vi "SaveImage.vi"(6 "x":dbl, 7 "error in (no error)":errorcluster, 8 "in path":path, 9 "Snap":bool, 10 "Image In":T1) -> (0 "error out":errorcluster)   [LabVIEW 2017]
uses:
  <vilib>/vision/Image Controls.llb/IMAQ Image.ctl
  <vilib>/vision/driver/IMAQdx.llb/IMAQdx Acquisition Mode.ctl
  <vilib>/vision/driver/NI_Vision_Acquisition_Software.lvlib
panel:
  out "Image":T1(plugin-control)
  out "number (0 to 1)":dbl
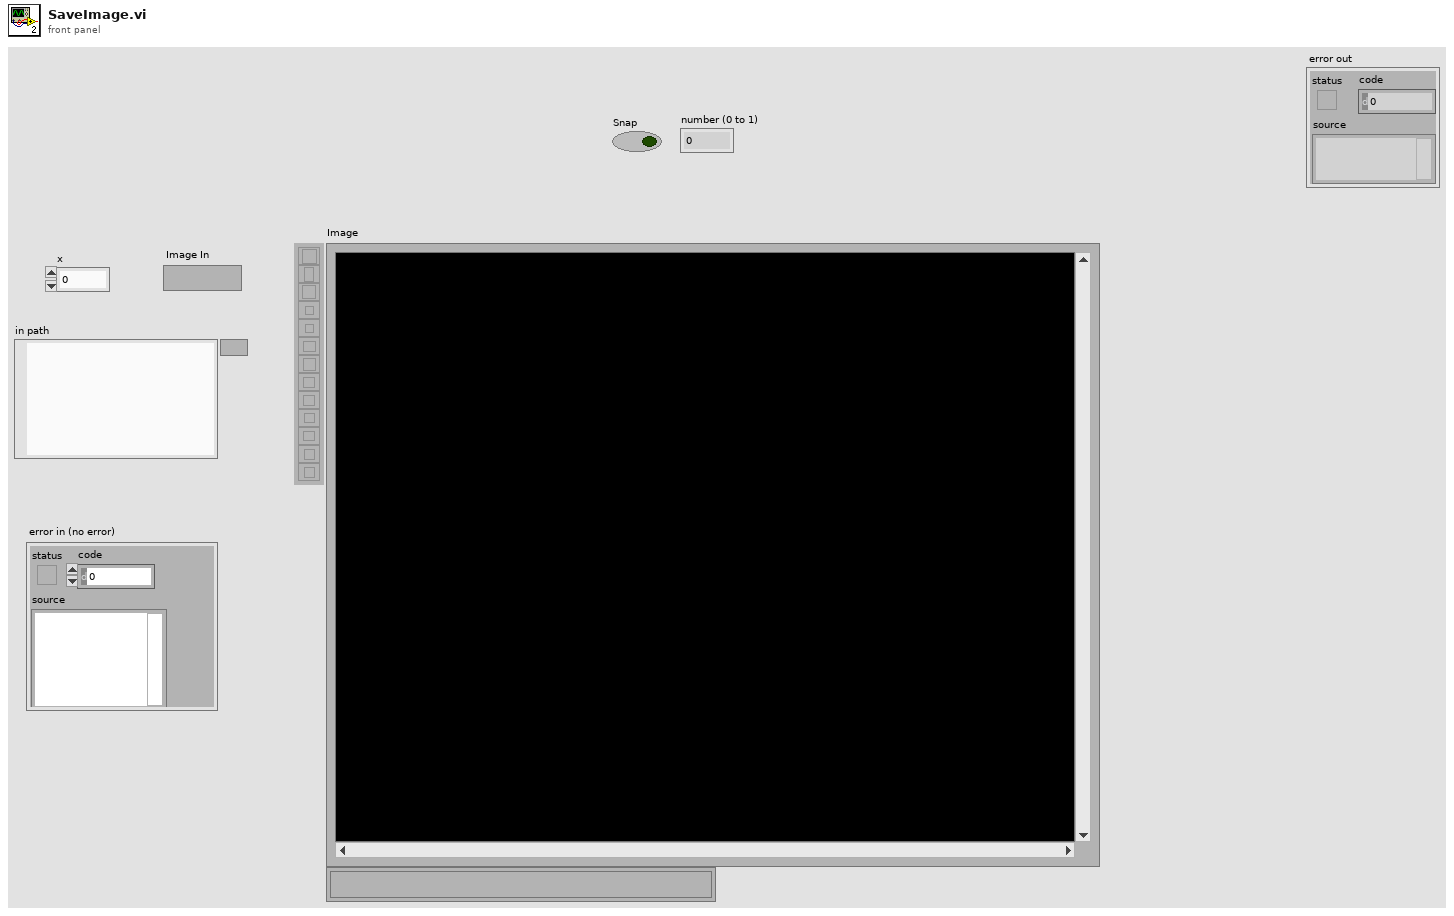
[diagram p1: front panel]
types:
  T1 = typedef "IMAQ Image.ctl" = refnum<image>
  T2 = typedef "NI_Vision_Acquisition_Software.lvlib/IMAQdx Acquisition Mode.ctl" = enum32{"One Shot", "Continuous"}
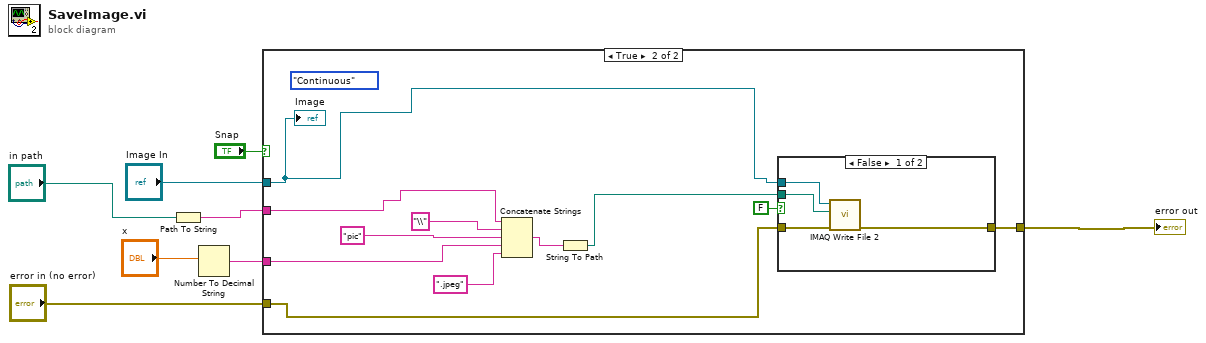
[diagram p0: block diagram]
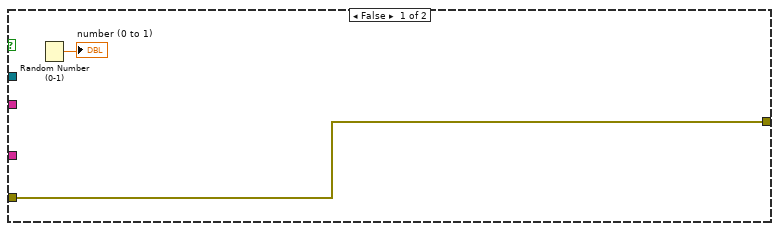
[diagram p2: hidden frame]
diagram:
  n1 = Path To String(path="in path") -> (string=w4:string)
  n2 = Number To Decimal String(number="x") -> (decimal integer string=w2:string)  [unwired: 1 in]
  n3 = case shown="True" "Snap" {
    tunnel: "Image In" -> [_ w19]
    tunnel: "error in (no error)" -> [w10 w20]
    tunnel: [w10 w21] -> w1
    tunnel: w4 -> [_ w17]
    tunnel: w2 -> [_ w12]
    frame False {
      n4 = Random Number (0-1)() -> (number: 0 to 1=→"number (0 to 1)":dbl)
    }
    frame True {
      (unwired) IMAQdx_Acquisition_Mode."Continuous" ("Continuous?")
      n5 = Concatenate Strings(w17, "\\" ("string"), "pic" ("string"), w12, ".jpeg" ("string")) -> (w15:string)
      n6 = String To Path(string=w15) -> (path=w14:path)
      n7 = case shown="False" FALSE {
        tunnel: w14 -> [w24 _]
        tunnel: w20 -> [w23 w26]
        tunnel: [w25 w26] -> w21
        tunnel: w19 -> [w22 _]
        frame False {
          n8 = call-poly "IMAQ Write File 2"("error in (no error)"=w23, "File Path"=w24, "Image"=w22) -> ("error out"=w25:errorcluster)  [unwired: 7 in, 1 out]
        }
        frame True {
        }
      }
      "Image" <- w19
    }
  }
  "error out" <- w1
